vi "Autonomous Independent.vi"   [LabVIEW 2015]
doc: "This VI is called when autonomous begins, and will automatically be terminated when autonomous ends. You can carry out timed or sensor driven robot movement independently without needing to return to the caller."
uses:
  <vilib>/Rock Robotics/WPI/Utilities/WPI_GetSetVariantRefNum.vi
  <vilib>/Rock Robotics/Network Tables/NT Read String.vi
  <vilib>/Rock Robotics/Network Tables/NT Write Numeric Array.vi
panel:
  # "Be sure to right-click and choose Data Operations>>Make Current Value default if you want to save the array values with the VI"
types:
  T1 = typedef "WPI_JoystickDevRef.ctl" = cluster{"Device":T2}
  T2 = typedef "WPI_JoystickDeviceEnum.ctl" = enum16{"USB 0", "USB 1", "USB 2", "USB 3", "USB 4", "USB 5"}
  T3 = typedef "WPI_RobotDriveDevRef.ctl" = cluster{"DevStatus":errorcluster, "Motors[]":T4[], "Square Inputs":bool, "Max Output":dbl}
  T4 = typedef "WPI_MotorControlDeviceRef.ctl" = cluster{"DeviceStatus":errorcluster, "Type":T5, "PWM":cluster{"PWM Channel":T6, "DeadBand":T7}, "CAN":cluster{"Device Number":u8, "Control Mode":T8, "Semaphore":T9, "Max Vout":dbl, "TalonSRX Control Mode":T10}, "Invert":bool}
  T5 = typedef "WPI_MotorControlType.ctl" = enum16{"PWM", "CAN", "CANTalonSRX"}
  T6 = typedef "FPGA_DIOPWMChannel.ctl" = enum8{"PWM 0", "PWM 1", "PWM 2", "PWM 3", "PWM 4", "PWM 5", "PWM 6", "PWM 7", "PWM 8", "PWM 9", "PWM MXP 0", "PWM MXP 1", "PWM MXP 2", "PWM MXP 3", "PWM MXP 4", "PWM MXP 5", "PWM MXP 6", "PWM MXP 7", "PWM MXP 8", "PWM MXP 9", "Invalid"}
  T7 = typedef "WPI_PWMDeadband.ctl" = cluster{"Name":string, "maxPositivePwm":i32, "minPositivePwm":i32, "centerPwm":i32, "maxNegativePwm":i32, "minNegativePwm":i32, "angularRange":u16}
  T8 = typedef "WPI_CANJaguar_ControlMode.ctl" = enum8{"Percent VBus", "Current", "Speed", "Position", "Voltage"}
  T9 = typedef "Semaphore RefNum" = refnum<k1>
  T10 = typedef "WPI_CANTalonSRX_APIControlMode.ctl" = enum8{"Percent VBus", "Speed", "Position", "Slave", "Unchanged / Invalid", "Voltage Compensation", "Current", "Motion Profile"}
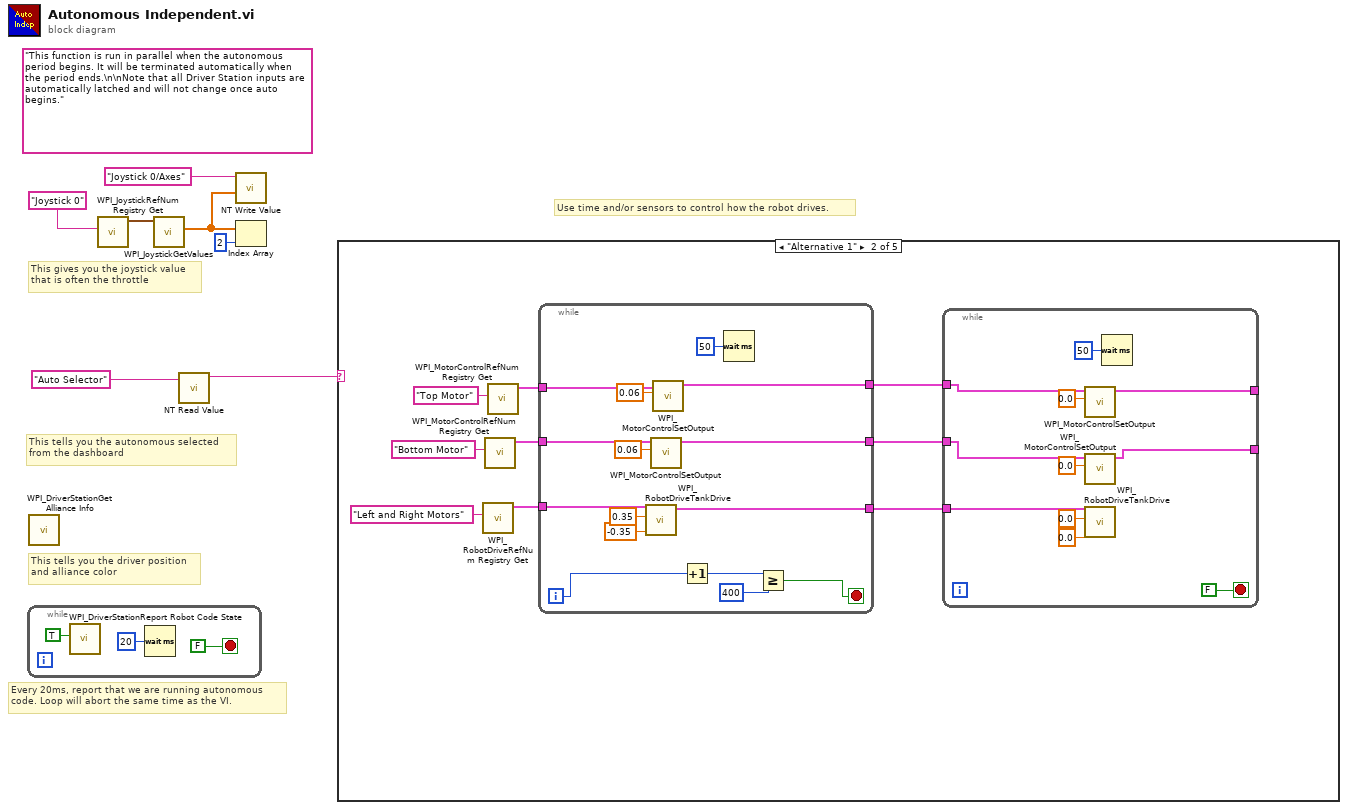
[diagram p0: block diagram]
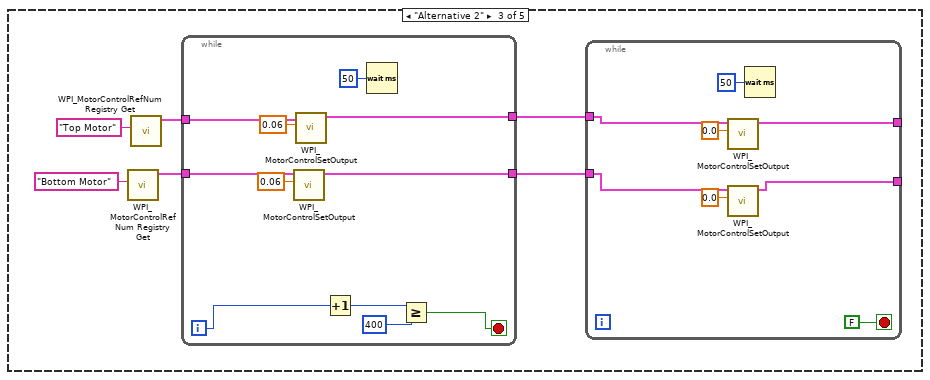
[diagram p3: hidden frame]
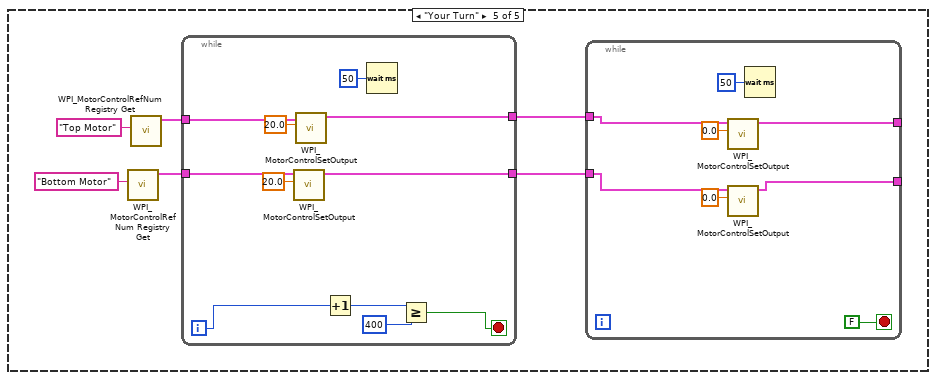
[diagram p5: hidden frame]
diagram:
  (unwired) "This function is run in parallel when the autonomous period begins. It will be terminated automatically when the period ends.\n\nNote that all Driver Station inputs are automatically latched and will not change once auto begins."
  # "This tells you the autonomous selected\nfrom the dashboard"
  # "Every 20ms, report that we are running autonomous\ncode. Loop will abort the same time as the VI."
  # "This gives you the joystick value\nthat is often the throttle"
  # "Use time and/or sensors to control how the robot drives."
  # "This tells you the driver position\nand alliance color"
  n1 = while {
    stop <- FALSE stop-if-true
    n2 = call <vilib>:"WPI_DriverStationReport Robot Code State.vi"("Autonomous"=TRUE) -> ()  [unwired: 10 in, 1 out]
    n3 = Wait (ms)(milliseconds to wait=u32 20) -> ()  [unwired: 1 out]
  }
  n4 = call <vilib>:"WPI_DriverStationGet Alliance Info.vi"() -> ()  [unwired: 12 out]
  n5 = call <vilib>:"WPI_JoystickRefNum Registry Get.vi"("refnum name"="Joystick 0") -> ("JoystickDevRef"=w6:T1)  [unwired: 1 in, 9 out]
  n6 = call <vilib>:"WPI_JoystickGetValues.vi"("JoystickDevRef"=w6) -> ("Axes"=w2:dbl[])  [unwired: 6 in, 4 out]
  n7 = call-poly <vilib>:"NT Read Value.vi"("Name"="Auto Selector") -> ("String"=w3:string)  [unwired: 9 in, 1 out]
  n8 = call-poly <vilib>:"NT Write Value.vi"("Numeric Array"=w2, "Name"="Joystick 0/Axes") -> ()  [unwired: 9 in, 1 out]
  n9 = Index Array(array=w2, index=2) -> ()  [unwired: 1 out]
  n10 = case shown="\"Alternative 1\"" w3 {
    frame Default {
      # "You can put your main auto here, or you can right-click on the case and make any\nother frame be the default case."
      # "This is the frame that will execute if no selection is made, or if it is not recognized"
    }
    frame "Alternative 1" {
      n11 = call <vilib>:"WPI_RobotDriveRefNum Registry Get.vi"("refnum name"="Left and Right Motors") -> ("RobotDriveDevRef"=w13:T3)  [unwired: 9 in, 1 out]
      n12 = call <vilib>:"WPI_MotorControlRefNum Registry Get.vi"("refnum name"="Bottom Motor") -> ("MotorControlDevRef"=w14:T4)  [unwired: 9 in, 1 out]
      n13 = call <vilib>:"WPI_MotorControlRefNum Registry Get.vi"("refnum name"="Top Motor") -> ("MotorControlDevRef"=w15:T4)  [unwired: 9 in, 1 out]
      n14 = while {
        tunnel: w14 -> [w45]
        tunnel: w15 -> [w44]
        tunnel: [w38] -> w18
        tunnel: [w37] -> w19
        tunnel: w13 -> [w34]
        tunnel: [w33] -> w12
        i -> [w40]
        stop <- w41 stop-if-true
        n15 = call <vilib>:"WPI_RobotDriveTankDrive.vi"("Right axis value"=-0.35, "Left axis value"=0.35, "RobotDriveDevRef"=w34) -> ("RobotDriveDevRef"=w33:T3)  [unwired: 6 in, 2 out]
        n16 = call <vilib>:"WPI_MotorControlSetOutput.vi"("Output"=0.06, "MotorControlDevRef"=w45) -> ("MotorControlDevRef"=w37:T4)  [unwired: 7 in, 2 out]
        n17 = call <vilib>:"WPI_MotorControlSetOutput.vi"("Output"=0.06, "MotorControlDevRef"=w44) -> ("MotorControlDevRef"=w38:T4)  [unwired: 7 in, 2 out]
        n18 = Increment(x=w40) -> (x+1=w42:i32)
        n19 = Wait (ms)(milliseconds to wait=u32 50) -> ()  [unwired: 1 out]
        n20 = Greater Or Equal?(x=w42, y=400) -> (x >= y?=w41:bool)
      }
      n21 = while {
        tunnel: w18 -> [w28]
        tunnel: w19 -> [w26]
        tunnel: [w27] -> _
        tunnel: [w25] -> _
        tunnel: w12 -> [w22]
        stop <- FALSE stop-if-true
        n22 = call <vilib>:"WPI_MotorControlSetOutput.vi"("Output"=0.0, "MotorControlDevRef"=w28) -> ("MotorControlDevRef"=w27:T4)  [unwired: 7 in, 2 out]
        n23 = call <vilib>:"WPI_MotorControlSetOutput.vi"("Output"=0.0, "MotorControlDevRef"=w26) -> ("MotorControlDevRef"=w25:T4)  [unwired: 7 in, 2 out]
        n24 = call <vilib>:"WPI_RobotDriveTankDrive.vi"("Right axis value"=0.0, "Left axis value"=0.0, "RobotDriveDevRef"=w22) -> ()  [unwired: 6 in, 3 out]
        n25 = Wait (ms)(milliseconds to wait=u32 50) -> ()  [unwired: 1 out]
      }
    }
    frame "Alternative 2" {
      n26 = call <vilib>:"WPI_MotorControlRefNum Registry Get.vi"("refnum name"="Bottom Motor") -> ("MotorControlDevRef"=w51:T4)  [unwired: 9 in, 1 out]
      n27 = call <vilib>:"WPI_MotorControlRefNum Registry Get.vi"("refnum name"="Top Motor") -> ("MotorControlDevRef"=w50:T4)  [unwired: 9 in, 1 out]
      n28 = while {
        tunnel: w51 -> [w70]
        tunnel: w50 -> [w69]
        tunnel: [w63] -> w47
        tunnel: [w62] -> w46
        i -> [w65]
        stop <- w66 stop-if-true
        n29 = call <vilib>:"WPI_MotorControlSetOutput.vi"("Output"=0.06, "MotorControlDevRef"=w70) -> ("MotorControlDevRef"=w62:T4)  [unwired: 7 in, 2 out]
        n30 = call <vilib>:"WPI_MotorControlSetOutput.vi"("Output"=0.06, "MotorControlDevRef"=w69) -> ("MotorControlDevRef"=w63:T4)  [unwired: 7 in, 2 out]
        n31 = Increment(x=w65) -> (x+1=w67:i32)
        n32 = Wait (ms)(milliseconds to wait=u32 50) -> ()  [unwired: 1 out]
        n33 = Greater Or Equal?(x=w67, y=400) -> (x >= y?=w66:bool)
      }
      n34 = while {
        tunnel: w47 -> [w57]
        tunnel: w46 -> [w55]
        tunnel: [w56] -> _
        tunnel: [w54] -> _
        stop <- FALSE stop-if-true
        n35 = call <vilib>:"WPI_MotorControlSetOutput.vi"("Output"=0.0, "MotorControlDevRef"=w57) -> ("MotorControlDevRef"=w56:T4)  [unwired: 7 in, 2 out]
        n36 = call <vilib>:"WPI_MotorControlSetOutput.vi"("Output"=0.0, "MotorControlDevRef"=w55) -> ("MotorControlDevRef"=w54:T4)  [unwired: 7 in, 2 out]
        n37 = Wait (ms)(milliseconds to wait=u32 50) -> ()  [unwired: 1 out]
      }
    }
    frame "Alternative 3" {
    }
    frame "Your Turn" {
      n38 = call <vilib>:"WPI_MotorControlRefNum Registry Get.vi"("refnum name"="Bottom Motor") -> ("MotorControlDevRef"=w76:T4)  [unwired: 9 in, 1 out]
      n39 = call <vilib>:"WPI_MotorControlRefNum Registry Get.vi"("refnum name"="Top Motor") -> ("MotorControlDevRef"=w75:T4)  [unwired: 9 in, 1 out]
      n40 = while {
        tunnel: w76 -> [w95]
        tunnel: w75 -> [w94]
        tunnel: [w88] -> w72
        tunnel: [w87] -> w71
        i -> [w90]
        stop <- w91 stop-if-true
        n41 = call <vilib>:"WPI_MotorControlSetOutput.vi"("Output"=20.0, "MotorControlDevRef"=w95) -> ("MotorControlDevRef"=w87:T4)  [unwired: 7 in, 2 out]
        n42 = call <vilib>:"WPI_MotorControlSetOutput.vi"("Output"=20.0, "MotorControlDevRef"=w94) -> ("MotorControlDevRef"=w88:T4)  [unwired: 7 in, 2 out]
        n43 = Increment(x=w90) -> (x+1=w92:i32)
        n44 = Wait (ms)(milliseconds to wait=u32 50) -> ()  [unwired: 1 out]
        n45 = Greater Or Equal?(x=w92, y=400) -> (x >= y?=w91:bool)
      }
      n46 = while {
        tunnel: w72 -> [w82]
        tunnel: w71 -> [w80]
        tunnel: [w81] -> _
        tunnel: [w79] -> _
        stop <- FALSE stop-if-true
        n47 = call <vilib>:"WPI_MotorControlSetOutput.vi"("Output"=0.0, "MotorControlDevRef"=w82) -> ("MotorControlDevRef"=w81:T4)  [unwired: 7 in, 2 out]
        n48 = call <vilib>:"WPI_MotorControlSetOutput.vi"("Output"=0.0, "MotorControlDevRef"=w80) -> ("MotorControlDevRef"=w79:T4)  [unwired: 7 in, 2 out]
        n49 = Wait (ms)(milliseconds to wait=u32 50) -> ()  [unwired: 1 out]
      }
    }
  }
